vi "Create ISO 8601 File Name.vi"(6 "File Extension":string="csv", 7 "Start Time Stamp":timestamp, 8 "Error In":errorcluster, 11 "Log Folder":path) -> (0 "Error Out":errorcluster, 3 "ISO 8601 File":path)   [LabVIEW 2017, in "Logger.lvlib" / "File.lvlib"]
uses:
  File.lvlib
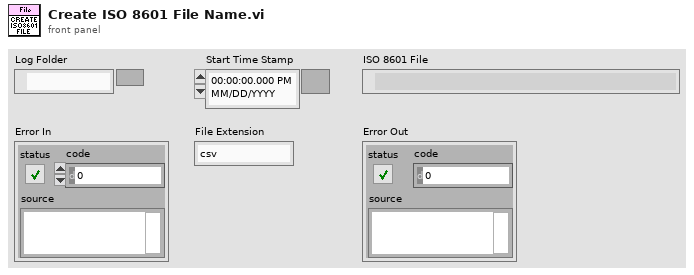
[diagram p1: front panel]
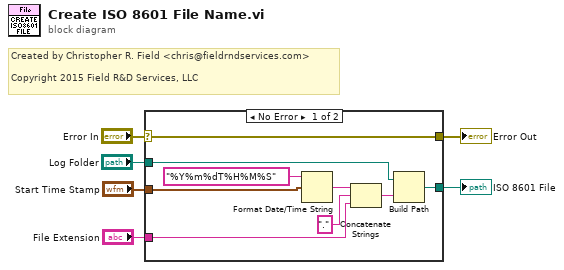
[diagram p0: block diagram]
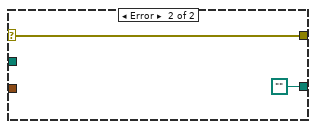
[diagram p2: hidden frame]
diagram:
  # "Created by Christopher R. Field <chris@fieldrndservices.com>\n\nCopyright 2015 Field R&D Services, LLC"
  n1 = case shown="No Error" "Error In" {
    selector: "Error In" -> [w8 w17]
    tunnel: "Start Time Stamp" -> [w11 _]
    tunnel: "Log Folder" -> [w10 _]
    tunnel: [w9 path ""] -> w3
    tunnel: [w8 w17] -> w2
    tunnel: "File Extension" -> [w7 _]
    frame No Error {
      n2 = Format Date/Time String(time format string (%c)="%Y%m%dT%H%M%S", seconds (now)=w11) -> (date/time string=w14:string)  [unwired: 1 in]
      n3 = Concatenate Strings(w14, "." ("string"), w7) -> (w12:string)
      n4 = Build Path(base path=w10, name or relative path=w12) -> (appended path=w9:path)
    }
    frame Error {
    }
  }
  "ISO 8601 File" <- w3
  "Error Out" <- w2
